vi "signalGenerator.vi"(8 "error in":errorcluster, 10 "cnt":T1, 11 "Square Wave":T2) -> (0 "error out":errorcluster, 3 "signal out_display":waveform(dbl))   [LabVIEW 2019]
uses:
  Set_AO_Wave-config.ctl
  type_signal.ctl
  _ctrl/rw.ctl
  <vilib>/measure/NI_MABase.lvlib
panel:
  out "Waveform Graph":waveform(dbl)(graph)
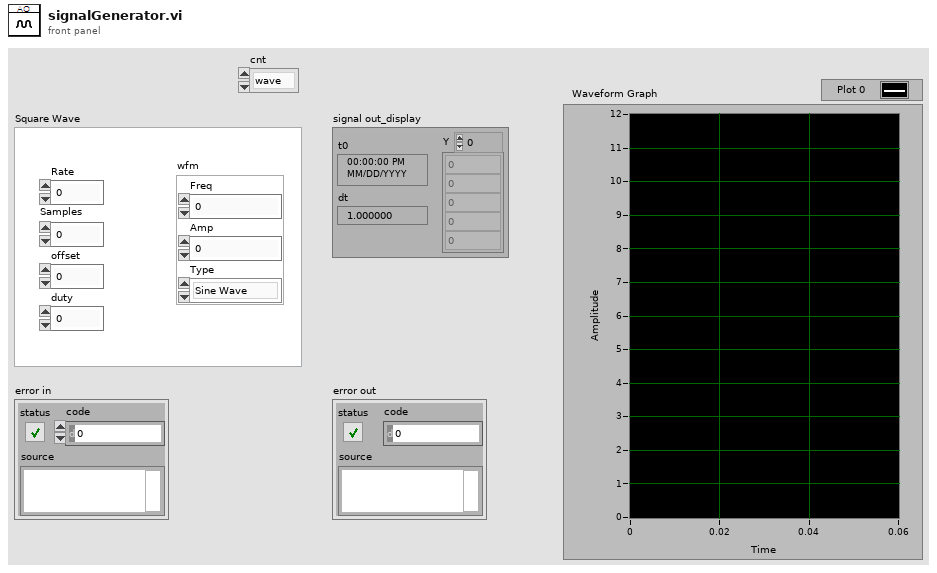
[diagram p1: front panel]
types:
  T1 = typedef "type_signal.ctl" = enum16{"wave", "level"}
  T2 = typedef "Set_AO_Wave-config.ctl" = cluster{"offset":dbl, "Samples":i32, "duty":dbl, "Rate":dbl, "wfm":cluster{"Freq":dbl, "Amp":dbl, "Type":enum16{"Sine Wave", "Triangle Wave", "Square Wave", "Sawtooth Wave"}}}
  T3 = typedef "rw.ctl" = enum16{"read", "write"}
  T4 = cluster{"Freq":dbl, "Amp":dbl, "Type":enum16{"Sine Wave", "Triangle Wave", "Square Wave", "Sawtooth Wave"}}
  T5 = enum16{"Sine Wave", "Triangle Wave", "Square Wave", "Sawtooth Wave"}
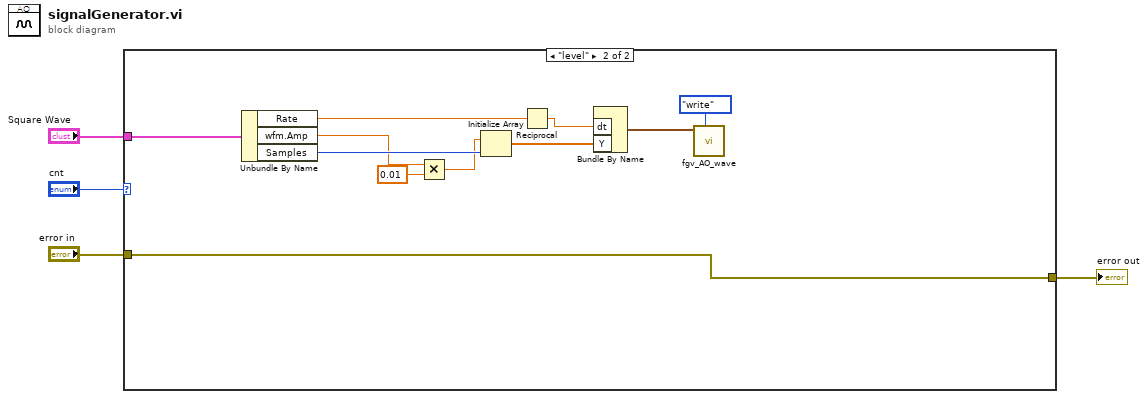
[diagram p0: block diagram]
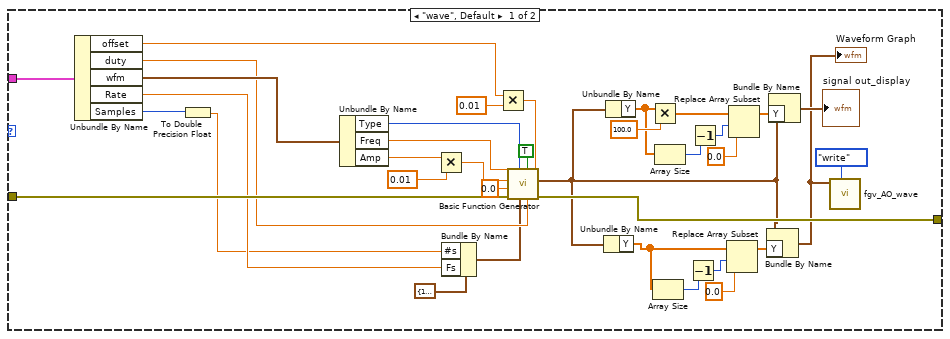
[diagram p2: hidden frame]
diagram:
  n1 = case shown="\"level\"" "cnt" {
    tunnel: "error in" -> [w40 w44]
    tunnel: [w39 w44] -> w3
    tunnel: "Square Wave" -> [w28 w51]
    frame "wave", Default {
      n2 = Unbundle By Name(w28) -> ("offset"=w26:dbl, "duty"=w25:dbl, "wfm"=w27:T4, "Rate"=w24:dbl, "Samples"=w22:i32)
      n3 = To Double Precision Float(number=w22) -> (double precision float=w21:dbl)
      n4 = Unbundle By Name(w27) -> ("Type"=w30:T5, "Freq"=w31:dbl, "Amp"=w32:dbl)
      n5 = Multiply(x=w32, y=0.01) -> (x*y=w34:dbl)
      n6 = Bundle By Name(cluster=cluster{"Fs":dbl, "#s":dbl} {"Fs"=1000.0, "#s"=1000.0} ("sampling info"), "#s"=w21, "Fs"=w24) -> (w23:cluster{"Fs":dbl, "#s":dbl})
      n7 = Multiply(x=w26, y=0.01) -> (x*y=w36:dbl)
      n8 = call <vilib>:"Basic Function Generator.vi"("offset"=w36, "square wave duty cycle (%)"=w25, "reset signal"=TRUE, "sampling info"=w23, "signal type"=w30, "error in (no error)"=w40, "phase"=0.0, "amplitude"=w34, "frequency"=w31) -> ("error out"=w39:errorcluster, "signal out"=w5:waveform(dbl))  [unwired: 1 out]
      n9 = Unbundle By Name(w5) -> ("Y"=w7:dbl[])
      n10 = Unbundle By Name(w5) -> ("Y"=w15:dbl[])
      n11 = Multiply(x=w15, y=100.0) -> (x*y=w17:dbl[])
      n12 = Array Size(array=w7) -> (size(s)=w10:i32)
      n13 = Array Size(array=w15) -> (size(s)=w14:i32)
      n14 = Decrement(x=w10) -> (x-1=w9:i32)
      n15 = Decrement(x=w14) -> (x-1=w13:i32)
      n16 = Replace Array Subset(array=w7, new element=0.0 ("new element/subarray"), index=w9) -> (w11:dbl[])
      n17 = Replace Array Subset(array=w17, new element=0.0 ("new element/subarray"), index=w13) -> (w16:dbl[])
      n18 = Bundle By Name(cluster=w5, "Y"=w11) -> (w6:waveform(dbl))
      "Waveform Graph" <- w6
      n19 = Bundle By Name(cluster=w5, "Y"=w16) -> (→"signal out_display":waveform(dbl))
      n20 = call "fgv_AO_wave.vi"("cmd"=rw."write", "signal in"=w6) -> ()  [unwired: 8 in, 2 out]
    }
    frame "level" {
      n21 = Unbundle By Name(w51) -> ("Rate"=w47:dbl, "wfm.Amp"=w43:dbl, "Samples"=w49:i32)
      n22 = Multiply(x=w43, y=0.01) -> (x*y=w41:dbl)
      n23 = Initialize Array(w41, w49) -> (w48:dbl[])
      n24 = Reciprocal(x=w47) -> (1/x=w46:dbl)
      n25 = Bundle By Name("dt"=w46, "Y"=w48) -> (w45:waveform(dbl))  [unwired: 1 in]
      n26 = call "fgv_AO_wave.vi"("cmd"=rw."write", "signal in"=w45) -> ()  [unwired: 8 in, 2 out]
    }
  }
  "error out" <- w3
